vi "_FPGA_DDS_CycleAccumulator_version2.vi"(0 "ConjSize":u8, 1 "Conj.InitCyc*2^32":u32, 2 "ConjArr":cluster{"Ratio*2^15":u16, "CycleDiff":u64}[](array[cluster])=[{"Ratio*2^15"=0, "CycleDiff"=0}, {"Ratio*2^15"=0, "CycleDiff"=0}, {"Ratio*2^15"=0, "CycleDiff"=0}, {"Ratio*2^15"=0, "CycleDiff"=0}, {"Ratio*2^15"=0, "CycleDiff"=0}, {"Ratio*2^15"=0, "CycleDiff"=0}, {"Ratio*2^15"=0, "CycleDiff"=0}, {"Ratio*2^15"=0, "CycleDiff"=0}, {"Ratio*2^15"=0, "CycleDiff"=0}, {"Ratio*2^15"=0, "CycleDiff"=0}, {"Ratio*2^15"=0, "CycleDiff"=0}, {"Ratio*2^15"=0, "CycleDiff"=0}, {"Ratio*2^15"=0, "CycleDiff"=0}, {"Ratio*2^15"=0, "CycleDiff"=0}, {"Ratio*2^15"=0, "CycleDiff"=0}, {"Ratio*2^15"=0, "CycleDiff"=0}], 3 "Update_ConjArr_strobe":bool, 4 "DeCycle*2^32":u64, 5 "1/DeCyc*2^8":u32, 6 "Conj.Mode":bool=TRUE, 7 "SlowCycle":bool, 9 "Reset":bool, 11 "IniCycle":u32) -> (10 "LastConj_strobe?":bool, 12 "Updating ConjArr?":bool, 14 "Not Conj?":bool, 15 "Conj Index":u8, 16 "Cross Quadrant?":bool, 17 "Quadrant":fxp<+,2,2>, 18 "Cross Zero Phase?":bool, 19 "RFCycleOut":u64)   [LabVIEW 2018]
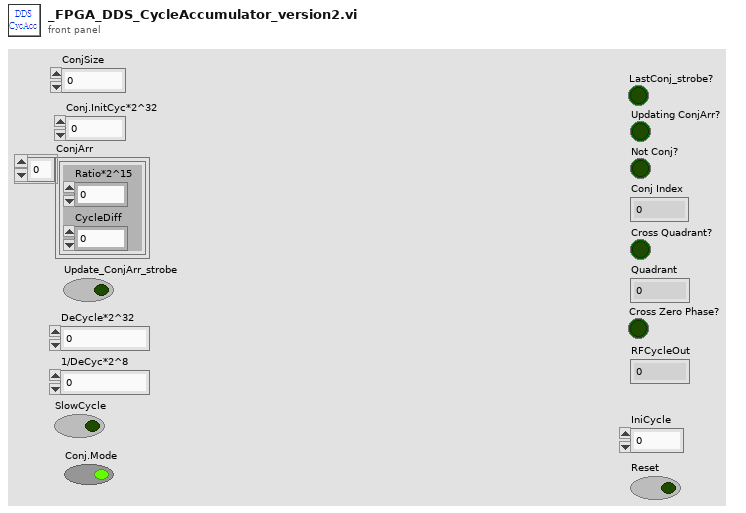
[diagram p1: front panel]
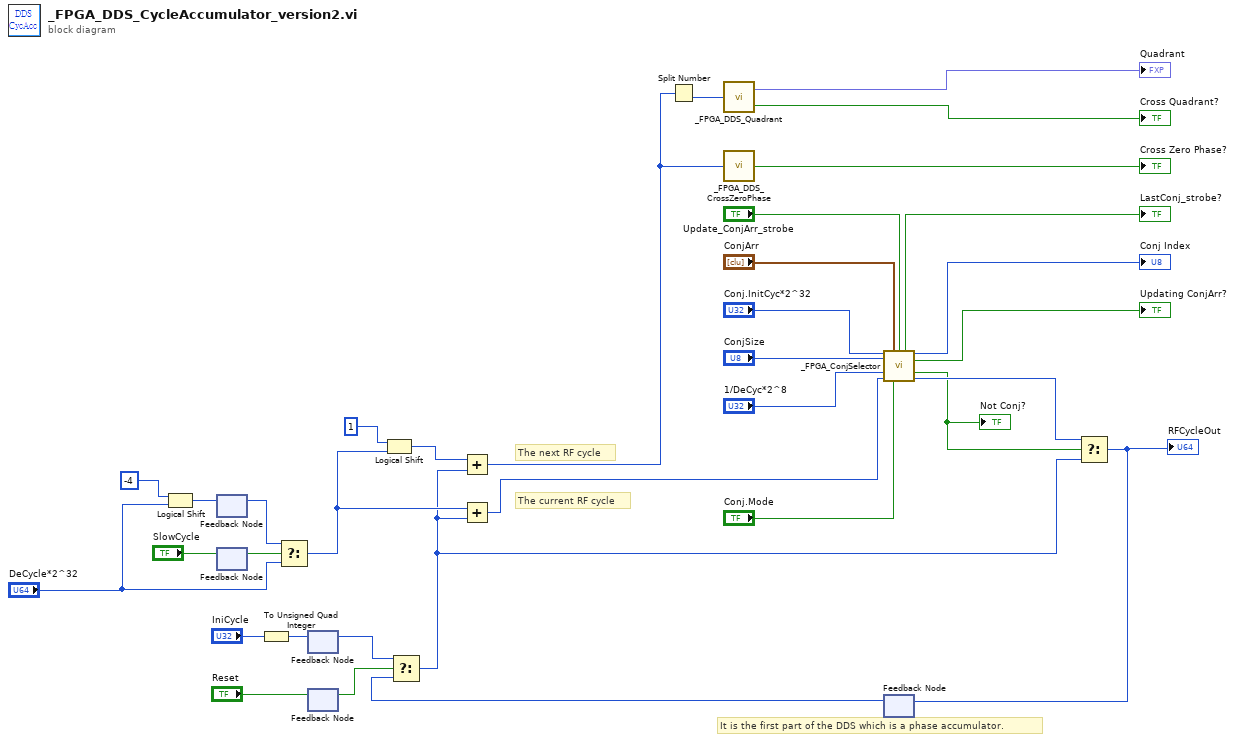
[diagram p0: block diagram]
diagram:
  # "It is the first part of the DDS which is a phase accumulator."
  # "The current RF cycle"
  # "The next RF cycle"
  n1 = Logical Shift(y=i16 -4 ("n"), x="DeCycle*2^32") -> (x << y=w33:u64)
  n2 = feedback-in #1(w33) -> ()
  n3 = feedback #1() -> (w31:u64)  [unwired: 1 in]
  n4 = feedback #2() -> (w29:bool)  [unwired: 1 in]
  n5 = feedback-in #2("SlowCycle") -> ()
  n6 = To Unsigned Quad Integer(1:"IniCycle") -> (0:w1:u64)
  n7 = Select(t=w31, s=w29, f="DeCycle*2^32") -> (s? t:f=w22:u64)
  n8 = feedback-in #3(w1) -> ()
  n9 = feedback #3() -> (w2:u64)  [unwired: 1 in]
  n10 = feedback #4() -> (w4:bool)  [unwired: 1 in]
  n11 = feedback-in #4("Reset") -> ()
  n12 = Logical Shift(y=i16 1 ("n"), x=w22) -> (x << y=w21:u64)
  n13 = feedback #5() -> (w7:u64)  [unwired: 1 in]
  n14 = Select(t=w2, s=w4, f=w7) -> (s? t:f=w6:u64)
  n15 = Add(x=w21, y=w6) -> (x+y=w16:u64)
  n16 = Add(x=w22, y=w6) -> (x+y=w20:u64)
  n17 = Split Number(x=w16) -> (lo(x)=w8:u32)  [unwired: 1 out]
  n18 = call "_FPGA_DDS_Quadrant.vi"("RfCyc_in"=w8) -> ("Cross?"=→"Cross Quadrant?":bool, "Quadrant"=→"Quadrant":fxp<+,2,2>)  [unwired: 2 in]
  n19 = call "_FPGA_DDS_CrossZeroPhase.vi"("RfCyc_in"=w16) -> ("Cross Zero Phase?"=→"Cross Zero Phase?":bool)
  n20 = call "_FPGA_ConjSelector.vi"("Conj.InitCyc*2^32"="Conj.InitCyc*2^32", "ConjArr"="ConjArr", "Init_strobe"="Update_ConjArr_strobe", "ConjSize-1"="ConjSize", "1/DeCyc*2^8"="1/DeCyc*2^8", "RfCyc_in"=w20, "Mode"="Conj.Mode") -> ("LastConj"=→"LastConj_strobe?":bool, "ConjIndex"=→"Conj Index":u8, "Initialising?"=→"Updating ConjArr?":bool, "Not Conj?"=w10:bool, "RfCyc_out"=w19:u64)  [unwired: 3 in, 1 out]
  "Not Conj?" <- w10
  n21 = Select(t=w19, s=w10, f=w6) -> (s? t:f=w18:u64)
  "RFCycleOut" <- w18
  n22 = feedback-in #5(w18) -> ()
